vi "3.0-FPGA FGtest.vi"() -> ()   [LabVIEW 2010]
panel:
  out "Has Refrence":bool
  in  "Enum":enum16{"Start", "End", "Borrow", "Return"}(ring)
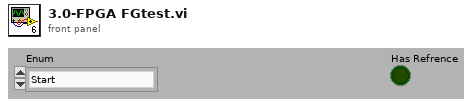
[diagram p1: front panel]
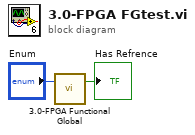
[diagram p0: block diagram]
diagram:
  n1 = call "3.0-FPGA Functional Global.vi"("Enum"="Enum") -> ("Has Refrence"=→"Has Refrence":bool)  [unwired: 1 in, 1 out]
